vi "CRYComplex Correction.vi"(7 "window":u16, 8 "Beta(relative record after zero pad.:0.5..1.0":dbl, 9 "Alpha(dev. from line freq.: -0.5..0.5 delta f)":dbl) -> (3 "Complex correction factor":cdb format="%.2f")   [LabVIEW 2013]
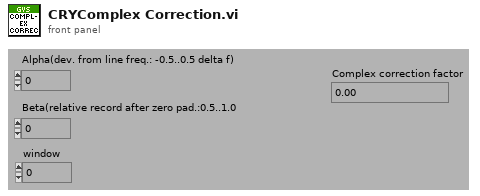
[diagram p1: front panel]
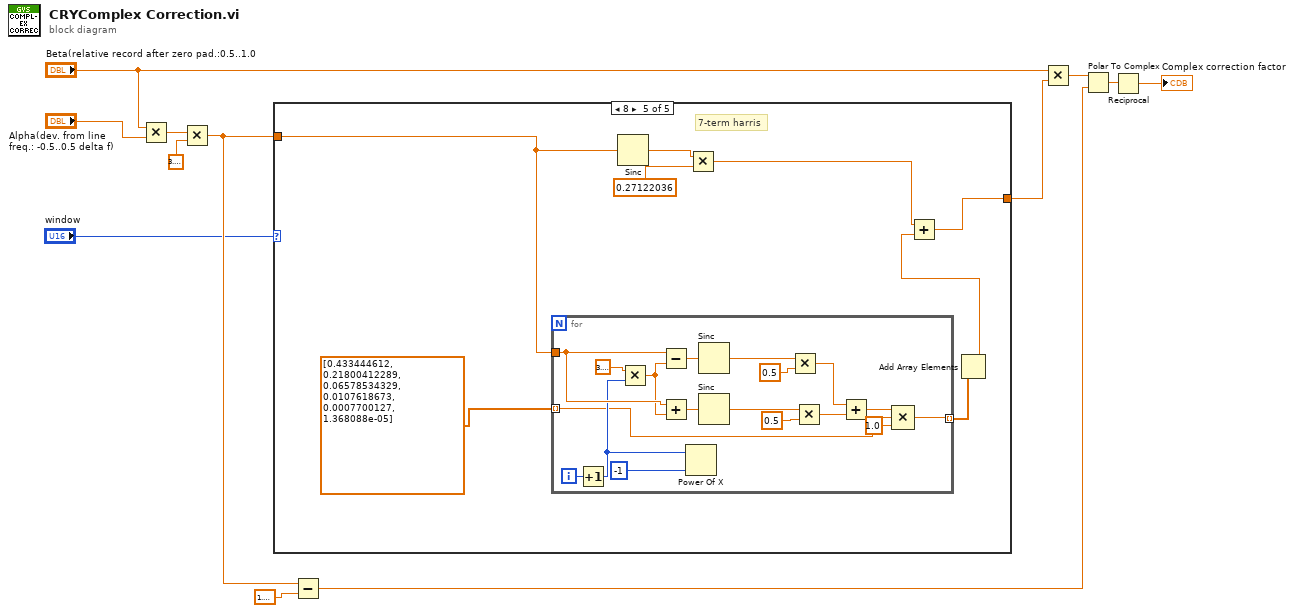
[diagram p0: block diagram]
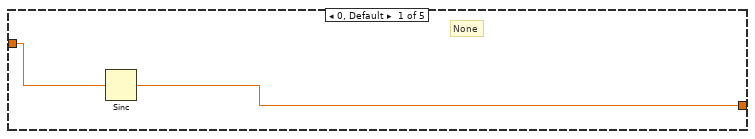
[diagram p2: hidden frame]
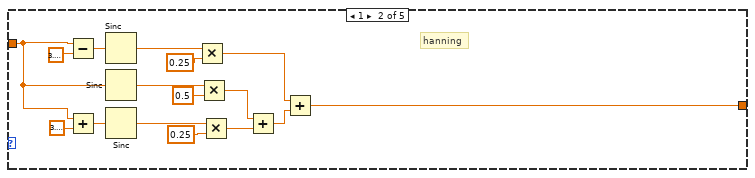
[diagram p3: hidden frame]
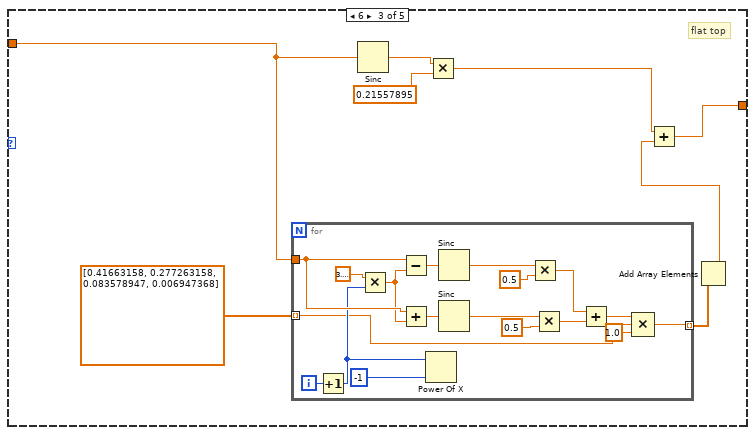
[diagram p4: hidden frame]
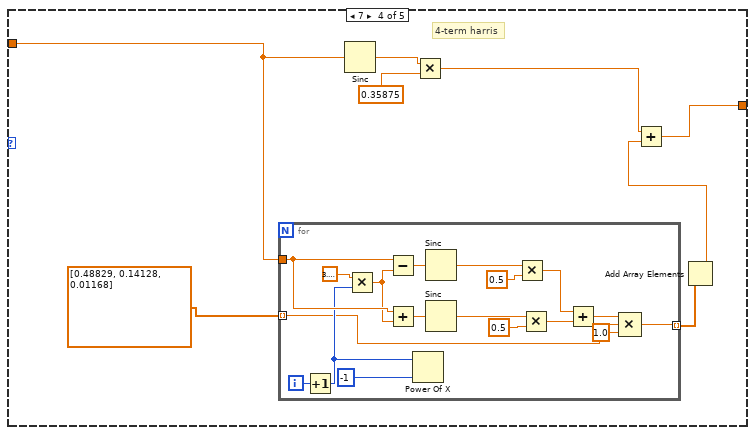
[diagram p5: hidden frame]
diagram:
  n1 = Multiply(x="Beta(relative record after zero pad.:0.5..1.0", y="Alpha(dev. from line freq.: -0.5..0.5 delta f)") -> (x*y=w4:dbl)
  n2 = Multiply(x=w4, y=3.141592653589793) -> (x*y=w3:dbl)
  n3 = case shown="8" "window" {
    tunnel: [w13 w26 w37 w58 w83] -> w12
    tunnel: w3 -> [w14 w22 w38 w57 w84]
    frame 0, Default {
      # "None"
      n4 = Sinc(1:w14) -> (0:w13:dbl)
    }
    frame 1 {
      # "hanning"
      n5 = Subtract(x=w22, y=3.141592653589793) -> (x-y=w23:dbl)
      n6 = Add(x=w22, y=3.141592653589793) -> (x+y=w15:dbl)
      n7 = Sinc(1:w23) -> (0:w20:dbl)
      n8 = Sinc(1:w22) -> (0:w21:dbl)
      n9 = Sinc(1:w15) -> (0:w16:dbl)
      n10 = Multiply(x=w20, y=0.25) -> (x*y=w28:dbl)
      n11 = Multiply(x=w21, y=0.5) -> (x*y=w29:dbl)
      n12 = Multiply(x=w16, y=0.25) -> (x*y=w30:dbl)
      n13 = Add(x=w29, y=w30) -> (x+y=w27:dbl)
      n14 = Add(x=w28, y=w27) -> (x+y=w26:dbl)
    }
    frame 6 {
      # "flat top"
      n15 = for {
        tunnel: w38 -> [w49]
        tunnel: dbl[] [0.41663158, 0.277263158, 0.083578947, 0.006947368] ("Array") -> [w41] mode=indexing
        tunnel: [w40] -> w33 mode=indexing
        i -> [w46]
        n16 = Increment(x=w46) -> (x+1=w43:i32)
        n17 = Multiply(x=3.141592653589793, y=w43) -> (x*y=w45:dbl)
        n18 = Subtract(x=w49, y=w45) -> (x-y=w55:dbl)
        n19 = Add(x=w49, y=w45) -> (x+y=w50:dbl)
        n20 = Power Of X(1:-1 ("y"), 2:w43) -> ()  [unwired: 1 out]
        n21 = Sinc(1:w55) -> (0:w54:dbl)
        n22 = Sinc(1:w50) -> (0:w51:dbl)
        n23 = Multiply(x=w54, y=0.5) -> (x*y=w48:dbl)
        n24 = Multiply(x=w51, y=0.5) -> (x*y=w56:dbl)
        n25 = Add(x=w48, y=w56) -> (x+y=w42:dbl)
        n26 = Compound Arithmetic op=MULTIPLY(w42, w41, 1.0 ("value")) -> (w40:dbl)
      }
      n27 = Sinc(1:w38) -> (0:w36:dbl)
      n28 = Multiply(x=w36, y=0.21557895) -> (x*y=w34:dbl)
      n29 = Add Array Elements(numeric array=w33) -> (sum=w32:dbl)
      n30 = Add(x=w34, y=w32) -> (x+y=w37:dbl)
    }
    frame 7 {
      # "4-term harris"
      n31 = for {
        tunnel: w57 -> [w75]
        tunnel: dbl[] [0.48829, 0.14128, 0.01168] ("Array") -> [w67] mode=indexing
        tunnel: [w66] -> w61 mode=indexing
        i -> [w72]
        n32 = Increment(x=w72) -> (x+1=w69:i32)
        n33 = Multiply(x=3.141592653589793, y=w69) -> (x*y=w71:dbl)
        n34 = Subtract(x=w75, y=w71) -> (x-y=w81:dbl)
        n35 = Add(x=w75, y=w71) -> (x+y=w76:dbl)
        n36 = Power Of X(1:-1 ("y"), 2:w69) -> ()  [unwired: 1 out]
        n37 = Sinc(1:w81) -> (0:w80:dbl)
        n38 = Sinc(1:w76) -> (0:w77:dbl)
        n39 = Multiply(x=w80, y=0.5) -> (x*y=w74:dbl)
        n40 = Multiply(x=w77, y=0.5) -> (x*y=w82:dbl)
        n41 = Add(x=w74, y=w82) -> (x+y=w68:dbl)
        n42 = Compound Arithmetic op=MULTIPLY(w68, w67, 1.0 ("value")) -> (w66:dbl)
      }
      n43 = Sinc(1:w57) -> (0:w64:dbl)
      n44 = Multiply(x=w64, y=0.35875) -> (x*y=w62:dbl)
      n45 = Add Array Elements(numeric array=w61) -> (sum=w60:dbl)
      n46 = Add(x=w62, y=w60) -> (x+y=w58:dbl)
    }
    frame 8 {
      # "7-term harris"
      n47 = for {
        tunnel: w84 -> [w101]
        tunnel: dbl[] [0.433444612, 0.21800412289, 0.06578534329, 0.0107618673, 0.0007700127, 1.368088e-05] ("Array") -> [w93] mode=indexing
        tunnel: [w92] -> w87 mode=indexing
        i -> [w98]
        n48 = Increment(x=w98) -> (x+1=w95:i32)
        n49 = Multiply(x=3.141592653589793, y=w95) -> (x*y=w97:dbl)
        n50 = Subtract(x=w101, y=w97) -> (x-y=w107:dbl)
        n51 = Add(x=w101, y=w97) -> (x+y=w102:dbl)
        n52 = Power Of X(1:-1 ("y"), 2:w95) -> ()  [unwired: 1 out]
        n53 = Sinc(1:w107) -> (0:w106:dbl)
        n54 = Sinc(1:w102) -> (0:w103:dbl)
        n55 = Multiply(x=w106, y=0.5) -> (x*y=w100:dbl)
        n56 = Multiply(x=w103, y=0.5) -> (x*y=w108:dbl)
        n57 = Add(x=w100, y=w108) -> (x+y=w94:dbl)
        n58 = Compound Arithmetic op=MULTIPLY(w94, w93, 1.0 ("value")) -> (w92:dbl)
      }
      n59 = Sinc(1:w84) -> (0:w90:dbl)
      n60 = Multiply(x=w90, y=0.27122036) -> (x*y=w88:dbl)
      n61 = Add Array Elements(numeric array=w87) -> (sum=w86:dbl)
      n62 = Add(x=w88, y=w86) -> (x+y=w83:dbl)
    }
  }
  n63 = Subtract(x=w3, y=1.5707963267948966) -> (x-y=w10:dbl)
  n64 = Multiply(x="Beta(relative record after zero pad.:0.5..1.0", y=w12) -> (x*y=w11:dbl)
  n65 = Polar To Complex(1:w10, 2:w11) -> (0:w9:cdb)
  n66 = Reciprocal(x=w9) -> (1/x=→"Complex correction factor":cdb)
